vi "Create waveform data type - 4 channels.vi"(8 "error in (no error)":errorcluster, 9 "Time Stamp":timestamp, 10 "sampling rate (Hz)":i32, 11 "scan data":dbl[](array[numeric])) -> (0 "error out":errorcluster, 1 "Channel 3":waveform(dbl), 2 "Channel 2":waveform(dbl), 5 "Channel 1":waveform(dbl), 7 "Channel 0":waveform(dbl))   [LabVIEW 2019, in "Main.lvclass"]
doc: "Developed by Kevin Thompson\nkevin@thompsonengineering.net\n\nCopyright 2020\nThompson Engineering, LLC"
uses:
  Main.lvclass
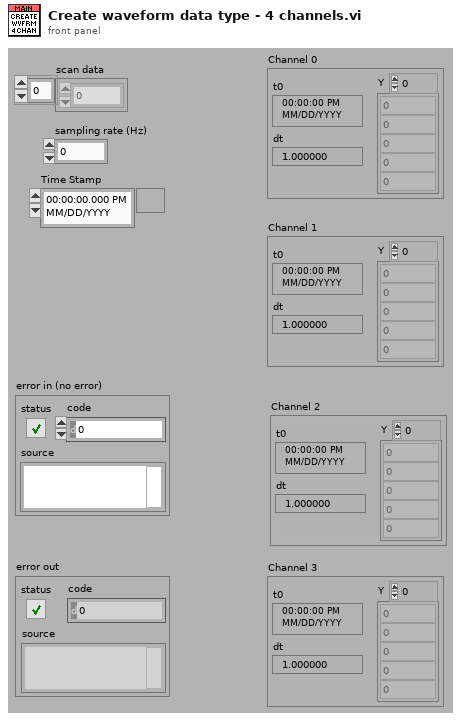
[diagram p1: front panel]
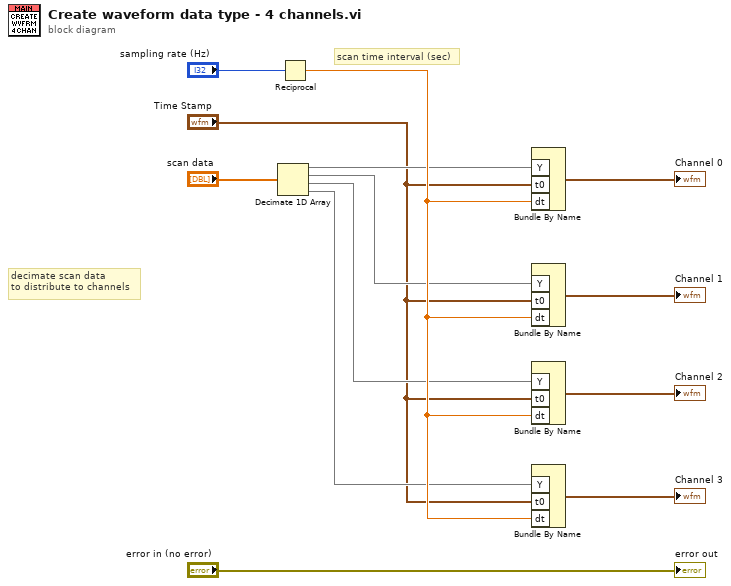
[diagram p0: block diagram]
diagram:
  # "scan time interval (sec)"
  # "decimate scan data\nto distribute to channels"
  n1 = Decimate 1D Array("scan data") -> (w6:dbl[], w5:dbl[], w4:dbl[], w3:dbl[])
  n2 = Reciprocal(x="sampling rate (Hz)") -> (1/x=w7:dbl)
  n3 = Bundle By Name("Y"=w6, "t0"="Time Stamp", "dt"=w7) -> (→"Channel 0":waveform(dbl))  [unwired: 1 in]
  n4 = Bundle By Name("Y"=w5, "t0"="Time Stamp", "dt"=w7) -> (→"Channel 1":waveform(dbl))  [unwired: 1 in]
  n5 = Bundle By Name("Y"=w4, "t0"="Time Stamp", "dt"=w7) -> (→"Channel 2":waveform(dbl))  [unwired: 1 in]
  n6 = Bundle By Name("Y"=w3, "t0"="Time Stamp", "dt"=w7) -> (→"Channel 3":waveform(dbl))  [unwired: 1 in]
  "error out" <- "error in (no error)"
